vi "setGlobals4.vi"() -> ()   [LabVIEW 2011]
panel:
  in  "Tab Control":enum32{"Page 1", "Page 2", "Page 3"}(tab)
  in  "Mass flow controllers":cluster{"MFC Range":u16, "MFC Name":string}[](array[cluster]) {"MFC Range" items=["0-10 sccm", "0-100 sccm", "0-1000 sccm"]}
  in  "D/A Cards":T1 {"Single-channel D/A (12-bit) Cards"."Channel 1" items=["N2 flow (NMFC1)", "H2 flow (HMFC1)", "Al2 flow (ALMFC1)", "Ga flow 1 (GAMFC1)", "Ga flow 2 (GAMFC2)", "Ga flow 3 (GAMFC3)", "In flow (INMFC1)", "P bubbler (PLMFC1)", "Plasma feed (ASLMFC1)", "P gas (PGMFC1)", "As gas (ASGMFC1)", "p-dopant flow 1 (PDOPMFC1)", "p-dopant flow 2 (PDOPMFC2)", "p-dopant flow 3 (PDOPMFC3)", "n-dopant flow 1 (NDOPMFC1)", "n-dopant flow 2 (NDOPMFC2)", "n-dopant flow 3 (PDOPMFC3)", "bad", "Fe flow 1 (FEMFC1)", "Fe flow 2 (FEMFC2)", "Fe flow 3 (FEMFC3)"]; "Quad D/A (10-bit) Cards"."Channel 4" items=["N2 flow (NMFC1)", "H2 flow (HMFC1)", "Al2 flow (ALMFC1)", "Ga flow 1 (GAMFC1)", "Ga flow 2 (GAMFC2)", "Ga flow 3 (GAMFC3)", "In flow (INMFC1)", "P bubbler (PLMFC1)", "Plasma feed (ASLMFC1)", "P gas (PGMFC1)", "As gas (ASGMFC1)", "p-dopant flow 1 (PDOPMFC1)", "p-dopant flow 2 (PDOPMFC2)", "p-dopant flow 3 (PDOPMFC3)", "n-dopant flow 1 (NDOPMFC1)", "n-dopant flow 2 (NDOPMFC2)", "n-dopant flow 3 (PDOPMFC3)", "bad", "Fe flow 1 (FEMFC1)", "Fe flow 2 (FEMFC2)", "Fe flow 3 (FEMFC3)"]; "Quad D/A (10-bit) Cards"."Channel 3" items=["N2 flow (NMFC1)", "H2 flow (HMFC1)", "Al2 flow (ALMFC1)", "Ga flow 1 (GAMFC1)", "Ga flow 2 (GAMFC2)", "Ga flow 3 (GAMFC3)", "In flow (INMFC1)", "P bubbler (PLMFC1)", "Plasma feed (ASLMFC1)", "P gas (PGMFC1)", "As gas (ASGMFC1)", "p-dopant flow 1 (PDOPMFC1)", "p-dopant flow 2 (PDOPMFC2)", "p-dopant flow 3 (PDOPMFC3)", "n-dopant flow 1 (NDOPMFC1)", "n-dopant flow 2 (NDOPMFC2)", "n-dopant flow 3 (PDOPMFC3)", "bad", "Fe flow 1 (FEMFC1)", "Fe flow 2 (FEMFC2)", "Fe flow 3 (FEMFC3)"]; "Quad D/A (10-bit) Cards"."Channel 2" items=["N2 flow (NMFC1)", "H2 flow (HMFC1)", "Al2 flow (ALMFC1)", "Ga flow 1 (GAMFC1)", "Ga flow 2 (GAMFC2)", "Ga flow 3 (GAMFC3)", "In flow (INMFC1)", "P bubbler (PLMFC1)", "Plasma feed (ASLMFC1)", "P gas (PGMFC1)", "As gas (ASGMFC1)", "p-dopant flow 1 (PDOPMFC1)", "p-dopant flow 2 (PDOPMFC2)", "p-dopant flow 3 (PDOPMFC3)", "n-dopant flow 1 (NDOPMFC1)", "n-dopant flow 2 (NDOPMFC2)", "n-dopant flow 3 (PDOPMFC3)", "bad", "Fe flow 1 (FEMFC1)", "Fe flow 2 (FEMFC2)", "Fe flow 3 (FEMFC3)"]; "Quad D/A (10-bit) Cards"."Channel 1" items=["N2 flow (NMFC1)", "H2 flow (HMFC1)", "Al2 flow (ALMFC1)", "Ga flow 1 (GAMFC1)", "Ga flow 2 (GAMFC2)", "Ga flow 3 (GAMFC3)", "In flow (INMFC1)", "P bubbler (PLMFC1)", "Plasma feed (ASLMFC1)", "P gas (PGMFC1)", "As gas (ASGMFC1)", "p-dopant flow 1 (PDOPMFC1)", "p-dopant flow 2 (PDOPMFC2)", "p-dopant flow 3 (PDOPMFC3)", "n-dopant flow 1 (NDOPMFC1)", "n-dopant flow 2 (NDOPMFC2)", "n-dopant flow 3 (PDOPMFC3)", "bad", "Fe flow 1 (FEMFC1)", "Fe flow 2 (FEMFC2)", "Fe flow 3 (FEMFC3)"]}
  out "output array":string[](array[string])
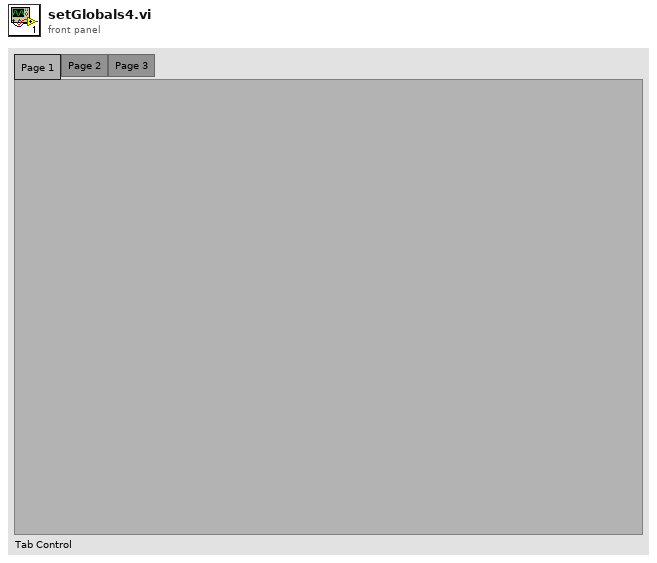
[diagram p1: front panel]
types:
  T1 = cluster{"Quad D/A (10-bit) Cards":cluster{"Channel 1":u16, "Channel 2":u16, "Channel 3":u16, "Channel 4":u16, "Name":string}[], "Single-channel D/A (12-bit) Cards":cluster{"Name":string, "Channel 1":u16}[]}
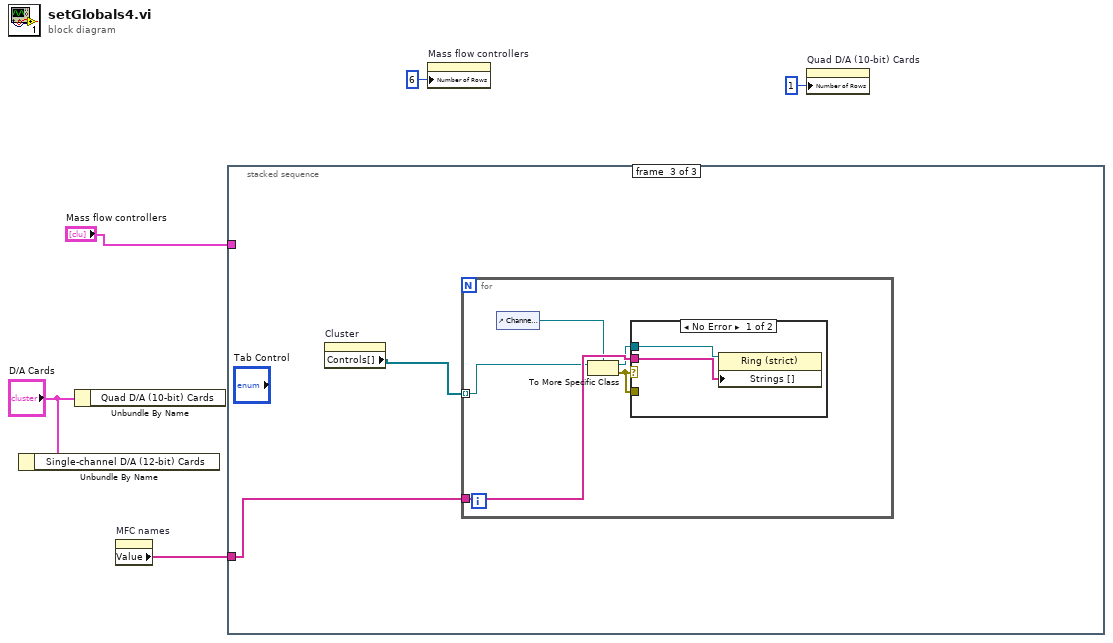
[diagram p0: block diagram]
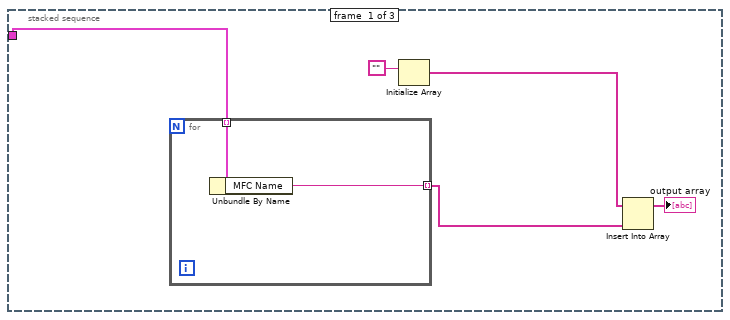
[diagram p2: hidden frame]
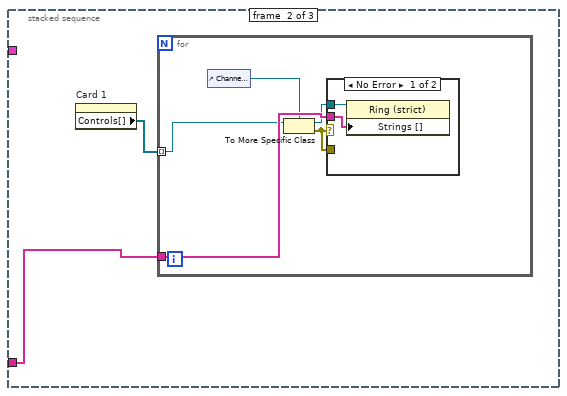
[diagram p3: hidden frame]
diagram:
  n1 = Unbundle By Name("D/A Cards") -> ()  [unwired: 1 out]
  n2 = Unbundle By Name("D/A Cards") -> ()  [unwired: 1 out]
  n3 = property on="MFC names" class="Arr (strict)"() -> ("Value"=w1:string[])  [unwired: 2 in, 2 out]
  n4 = stacked-sequence {
    tunnel: "Mass flow controllers" -> [w7 _ _]
    tunnel: w1 -> [_ w13 w22]
    frame #0 {
      n5 = for {
        tunnel: w7 -> [w12] mode=indexing
        tunnel: [w11] -> w9 mode=indexing
        n6 = Unbundle By Name(w12) -> ("MFC Name"=w11:string)
      }
      n7 = Initialize Array("") -> (w8:string[])  [unwired: 1 in]
      n8 = Insert Into Array(array=w8, new element=w9) -> (→"output array":string[])  [unwired: 1 in]
    }
    frame #1 {
      n9 = property on="Card 1" class="Clust (strict)"() -> ("Controls[]"=w14:refnum<vi>[])  [unwired: 2 in, 2 out]
      n10 = for {
        tunnel: w14 -> [w16] mode=indexing
        tunnel: w13 -> [w19]
        n11 = control-ref of="Channel 1"() -> (w15:refnum<vi>)
        n12 = To More Specific Class(target class=w15, reference=w16) -> (specific class reference=w18:refnum<vi>, error out=w17:errorcluster)  [unwired: 1 in]
        n13 = case shown="No Error" w17 {
          tunnel: w18 -> [w21 _]
          tunnel: w17 -> [_ _]
          tunnel: w19 -> [w20 _]
          frame No Error {
            n14 = property class="Ring (strict)"(reference=w21, "Strings []"=w20) -> ()  [unwired: 1 in, 2 out]
          }
          frame Error {
          }
        }
      }
    }
    frame #2 {
      n15 = property on="Cluster" class="Clust (strict)"() -> ("Controls[]"=w23:refnum<vi>[])  [unwired: 2 in, 2 out]
      n16 = for {
        tunnel: w23 -> [w25] mode=indexing
        tunnel: w22 -> [w28]
        n17 = control-ref of="Channel 1"() -> (w24:refnum<vi>)
        n18 = To More Specific Class(target class=w24, reference=w25) -> (specific class reference=w27:refnum<vi>, error out=w26:errorcluster)  [unwired: 1 in]
        n19 = case shown="No Error" w26 {
          tunnel: w27 -> [w29 _]
          tunnel: w26 -> [_ _]
          tunnel: w28 -> [w30 _]
          frame No Error {
            n20 = property class="Ring (strict)"(reference=w29, "Strings []"=w30) -> ()  [unwired: 1 in, 2 out]
          }
          frame Error {
          }
        }
      }
    }
  }
  n21 = property on="Mass flow controllers" class="Arr (strict)"("Number of Rows"=u32 6) -> ()  [unwired: 2 in, 2 out]
  n22 = property on="Quad D/A (10-bit) Cards" class="Arr (strict)"("Number of Rows"=u32 1) -> ()  [unwired: 2 in, 2 out]
